vi "Get UNIX Time in Nanoseconds.vi"(10 "Time Stamp":timestamp format="%<%x %.3X>T") -> (2 "UNIX Time (ns)":u64)   [LabVIEW 2020]
uses:
  <vilib>/LabVIEW Open Source Project/Epoch Date & Time/epoch.UNIX/Epoch.UNIX.lvclass
  C:/Program Files (x86)/National Instruments/LabVIEW 2020/vi.lib/LabVIEW Open Source Project/Epoch Date & Time/epoch/Epoch.lvclass
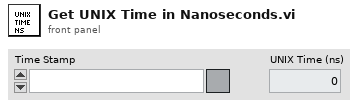
[diagram p1: front panel]
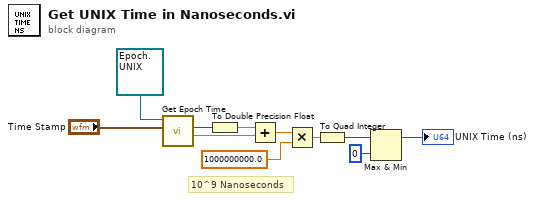
[diagram p0: block diagram]
diagram:
  # "10^9 Nanoseconds"
  n1 = call <vilib>:"Get Epoch Time.vi"("Timestamp (now)"="Time Stamp", "Epoch (Local)"=refnum<class "Epoch.UNIX.lvclass"> refnum ("Epoch.UNIX.lvclass")) -> ("Fractional Second"=w8:dbl, "Epoch Time (s)"=w9:i64)  [unwired: 7 in, 1 out]
  n2 = To Double Precision Float(number=w9) -> (double precision float=w5:dbl)
  n3 = Add(x=w5, y=w8) -> (x+y=w7:dbl)
  n4 = Multiply(x=w7, y=1000000000.0) -> (x*y=w6:dbl)
  n5 = To Quad Integer(1:w6) -> (0:w4:i64)
  n6 = Max & Min(x=w4, y=i64 0) -> (max(x,y)=→"UNIX Time (ns)":i64)  [unwired: 1 out]
